vi "AlliGator Hide Path Drop Boxes.vi"(8 "Error In":errorcluster, 9 "Hide (F)/Show":bool, 11 "AlliGator Ctrl Refnums":T1) -> (0 "Error Out":errorcluster)   [LabVIEW 2021, in "AlliGator Action Engine.lvlib"]
uses:
  AlliGator Action Engine.lvlib
  AlliGator Ctrl Refnums.ctl
  AlliGator Other Ctrl Refnums.ctl
  AlliGator State Indicator.ctl
  AlliGator Main Window Tabs.ctl
  AlliGator Phasor Plot Ctrl Refnums.ctl
  AlliGator Phasor Graph Ctrl Refnums.ctl
  Phasor/Phasor Calibration Type.ctl
  AlliGator Dataset Ctrl Refnums.ctl
  AlliGator Displayed Image.ctl
  AlliGator Registered Events Ctrl Refnums.ctl
  AlliGator Image Histogram Control Refnums.ctl
  Histograms/Linear Histogram Options.ctl
  Histograms/Histogram Bin Option.ctl
  Histograms/Histogram Bin Position.ctl
  AlliGator Decay Fit Map Control Refnums.ctl
  Fits/IRF(X)PSED/Decay Fit Parameters & Derived Quantities List.ctl
  AlliGator GUI.lvlib
  AlliGator Source Image.lvlib
  Phasor/Phasor.lvlib
  Histograms/Histogram Window.lvlib
  Fits/Fits.lvlib
  AlliGator Decay Fit Parameter Map.lvlib
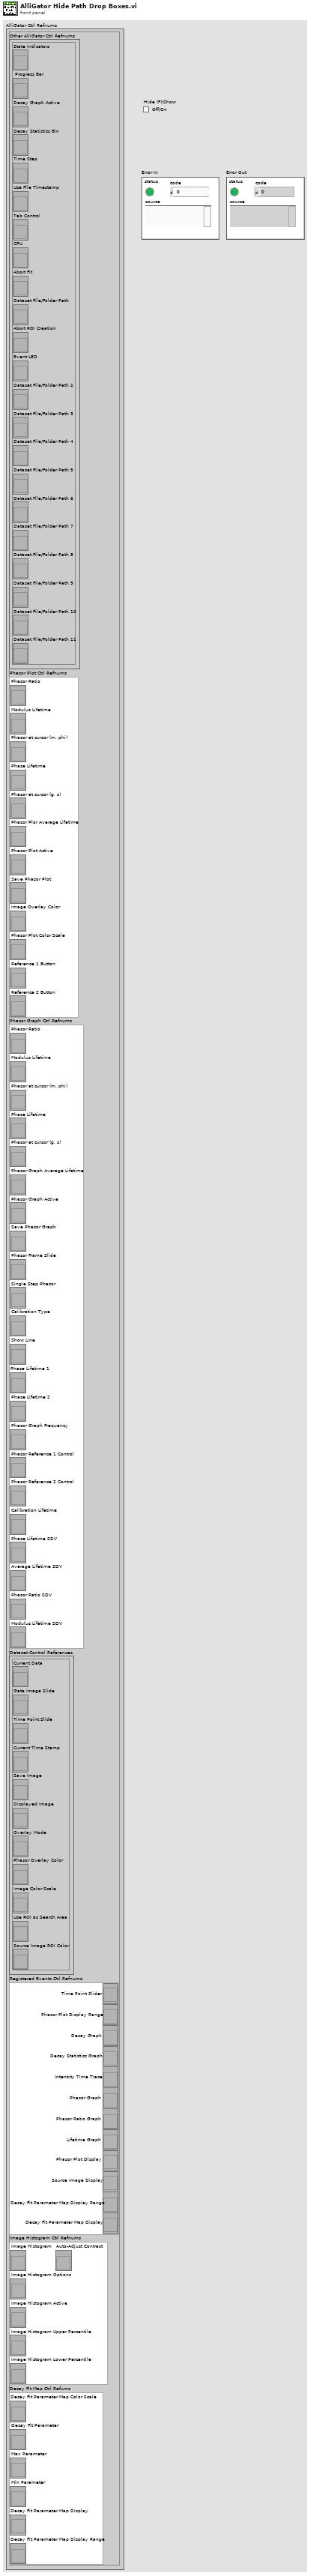
[diagram p1: front panel]
types:
  T1 = typedef "AlliGator GUI.lvlib/AlliGator Ctrl Refnums.ctl" = cluster{"Other AlliGator Ctrl Refnums":T2, "Phasor Plot Ctrl Refnums":T3, "Phasor Graph Ctrl Refnums":T4, "Dataset Control References":T5, "Registered Events Ctrl Refnums":T6, "Image Histogram Ctrl Refnums":T7, "Decay Fit Map Ctrl Refums":T8}
  T2 = typedef "AlliGator GUI.lvlib/AlliGator Other Ctrl Refnums.ctl" = cluster{"State Indicators":refnum<vi>, " Progress Bar":refnum<vi>, "Decay Graph Active":refnum<vi>, "Decay Statistics Bin":refnum<vi>, "Time Step":refnum<vi>, "Use File Timestamp":refnum<vi>, "Tab Control":refnum<vi>, "CPU":refnum<vi>, "Abort Fit":refnum<vi>, "Dataset File/Folder Path":refnum<vi>, "Abort ROI Creation":refnum<vi>, "Event LED":refnum<vi>, "Dataset File/Folder Path 2":refnum<vi>, "Dataset File/Folder Path 3":refnum<vi>, "Dataset File/Folder Path 4":refnum<vi>, "Dataset File/Folder Path 5":refnum<vi>, "Dataset File/Folder Path 6":refnum<vi>, "Dataset File/Folder Path 7":refnum<vi>, "Dataset File/Folder Path 8":refnum<vi>, "Dataset File/Folder Path 9":refnum<vi>, "Dataset File/Folder Path 10":refnum<vi>, "Dataset File/Folder Path 11":refnum<vi>}
  T3 = typedef "AlliGator GUI.lvlib/AlliGator Phasor Plot Ctrl Refnums.ctl" = cluster{"Phasor Ratio":refnum<vi>, "Modulus Lifetime":refnum<vi>, "Phasor at cursor (m, phi)":refnum<vi>, "Phase Lifetime":refnum<vi>, "Phasor at cursor (g, s)":refnum<vi>, "Phasor Plor Average Lifetime":refnum<vi>, "Phasor Plot Active":refnum<vi>, "Save Phasor Plot":refnum<vi>, "Image Overlay Color":refnum<vi>, "Phasor Plot Color Scale":refnum<vi>, "Reference 1 Button":refnum<vi>, "Reference 2 Button":refnum<vi>}
  T4 = typedef "AlliGator GUI.lvlib/AlliGator Phasor Graph Ctrl Refnums.ctl" = cluster{"Phasor Ratio":refnum<vi>, "Modulus Lifetime":refnum<vi>, "Phasor at cursor (m, phi)":refnum<vi>, "Phase Lifetime":refnum<vi>, "Phasor at cursor (g, s)":refnum<vi>, "Phasor Graph Average Lifetime":refnum<vi>, "Phasor Graph Active":refnum<vi>, "Save Phasor Graph":refnum<vi>, "Phasor Frame Slide":refnum<vi>, "Single Step Phasor":refnum<vi>, "Calibration Type":refnum<vi>, "Show Line":refnum<vi>, "Phase Lifetime 1":refnum<vi>, "Phase Lifetime 2":refnum<vi>, "Phasor Graph Frequency":refnum<vi>, "Phasor Reference 1 Control":refnum<vi>, "Phasor Reference 2 Control":refnum<vi>, "Calibration Lifetime":refnum<vi>, "Phase Lifetime SDV":refnum<vi>, "Average Lifetime SDV":refnum<vi>, "Phasor Ratio SDV":refnum<vi>, "Modulus Lifetime SDV":refnum<vi>}
  T5 = typedef "AlliGator GUI.lvlib/AlliGator Dataset Ctrl Refnums.ctl" = cluster{"Current Data":refnum<vi>, "Gate Image Slide":refnum<vi>, "Time Point Slide":refnum<vi>, "Current Time Stamp":refnum<vi>, "Save Image":refnum<vi>, "Displayed Image":refnum<vi>, "Overlay Mode":refnum<vi>, "Phasor Overlay Color":refnum<vi>, "Image Color Scale":refnum<vi>, "Use ROI as Search Area":refnum<vi>, "Source Image ROI Color":refnum<vi>}
  T6 = typedef "AlliGator GUI.lvlib/AlliGator Registered Events Ctrl Refnums.ctl" = cluster{"Time Point Slider":refnum<vi>, "Phasor Plot Display Range":refnum<vi>, "Decay Graph":refnum<vi>, "Decay Statistics Graph":refnum<vi>, "Intensity Time Trace":refnum<vi>, "Phasor Graph":refnum<vi>, "Phasor Ratio Graph":refnum<vi>, "Lifetime Graph":refnum<vi>, "Phasor Plot Display":refnum<vi>, "Source Image Display":refnum<vi>, "Decay Fit Parameter Map Display Range":refnum<vi>, "Decay Fit Parameter Map Display":refnum<vi>}
  T7 = typedef "AlliGator GUI.lvlib/AlliGator Image Histogram Control Refnums.ctl" = cluster{"Image Histogram":refnum<vi>, "Image Histogram Options":refnum<vi>, "Image Histogram Active":refnum<vi>, "Image Histogram Upper Percentile":refnum<vi>, "Image Histogram Lower Percentile":refnum<vi>, "Auto-Adjust Contrast":refnum<vi>}
  T8 = typedef "AlliGator Decay Fit Parameter Map.lvlib/AlliGator Decay Fit Map Control Refnums.ctl" = cluster{"Decay Fit Parameter Map Color Scale":refnum<vi>, "Decay Fit Parameter":refnum<vi>, "Max Parameter":refnum<vi>, "Min Parameter":refnum<vi>, "Decay Fit Parameter Map Display":refnum<vi>, "Decay Fit Parameter Map Display Range":refnum<vi>}
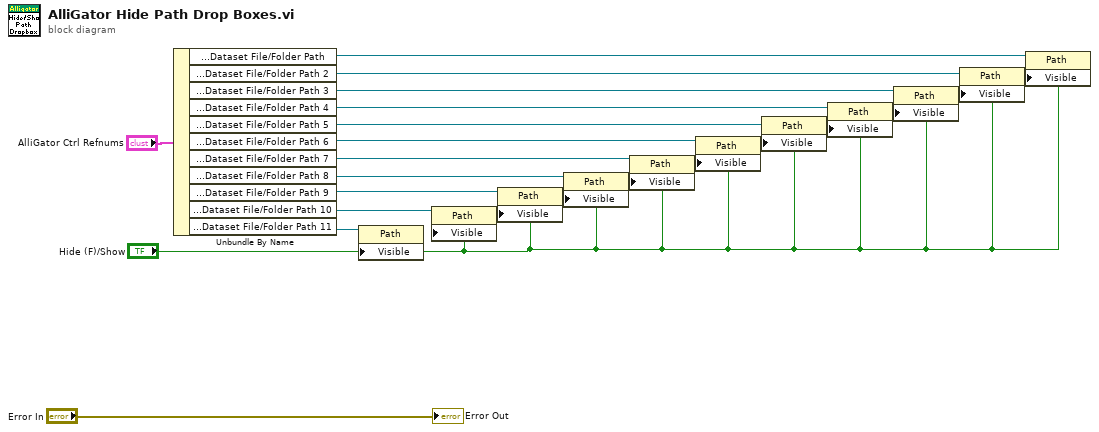
[diagram p0: block diagram]
diagram:
  n1 = Unbundle By Name("AlliGator Ctrl Refnums") -> ("Other AlliGator Ctrl Refnums.Dataset File/Folder Path"=w14:refnum<vi>, "Other AlliGator Ctrl Refnums.Dataset File/Folder Path 2"=w12:refnum<vi>, "Other AlliGator Ctrl Refnums.Dataset File/Folder Path 3"=w11:refnum<vi>, "Other AlliGator Ctrl Refnums.Dataset File/Folder Path 4"=w10:refnum<vi>, "Other AlliGator Ctrl Refnums.Dataset File/Folder Path 5"=w9:refnum<vi>, "Other AlliGator Ctrl Refnums.Dataset File/Folder Path 6"=w8:refnum<vi>, "Other AlliGator Ctrl Refnums.Dataset File/Folder Path 7"=w7:refnum<vi>, "Other AlliGator Ctrl Refnums.Dataset File/Folder Path 8"=w6:refnum<vi>, "Other AlliGator Ctrl Refnums.Dataset File/Folder Path 9"=w5:refnum<vi>, "Other AlliGator Ctrl Refnums.Dataset File/Folder Path 10"=w4:refnum<vi>, "Other AlliGator Ctrl Refnums.Dataset File/Folder Path 11"=w2:refnum<vi>)
  n2 = property class="Path"(reference=w2, "Visible"="Hide (F)/Show") -> ()  [unwired: 1 in, 2 out]
  n3 = property class="Path"(reference=w4, "Visible"="Hide (F)/Show") -> ()  [unwired: 1 in, 2 out]
  n4 = property class="Path"(reference=w5, "Visible"="Hide (F)/Show") -> ()  [unwired: 1 in, 2 out]
  n5 = property class="Path"(reference=w6, "Visible"="Hide (F)/Show") -> ()  [unwired: 1 in, 2 out]
  n6 = property class="Path"(reference=w7, "Visible"="Hide (F)/Show") -> ()  [unwired: 1 in, 2 out]
  n7 = property class="Path"(reference=w8, "Visible"="Hide (F)/Show") -> ()  [unwired: 1 in, 2 out]
  n8 = property class="Path"(reference=w9, "Visible"="Hide (F)/Show") -> ()  [unwired: 1 in, 2 out]
  n9 = property class="Path"(reference=w10, "Visible"="Hide (F)/Show") -> ()  [unwired: 1 in, 2 out]
  n10 = property class="Path"(reference=w11, "Visible"="Hide (F)/Show") -> ()  [unwired: 1 in, 2 out]
  n11 = property class="Path"(reference=w12, "Visible"="Hide (F)/Show") -> ()  [unwired: 1 in, 2 out]
  n12 = property class="Path"(reference=w14, "Visible"="Hide (F)/Show") -> ()  [unwired: 1 in, 2 out]
  "Error Out" <- "Error In"
